vi "Main VI.vi"(8 "error in":errorcluster) -> (0 "error out":errorcluster)   [LabVIEW 2023, in "Decoder.lvlib"]
uses:
  Decoder.lvlib
  <vilib>/xnet/xnet.llb/XNET Frame CAN.ctl
  <vilib>/xnet/xnet.llb/XNET Frame Type CAN.ctl
  <vilib>/xnet/xnet.llb/XNET Create Session (Frame Input Single-point).vi
  <vilib>/xnet/xnet.llb/XNET Read (Frame CAN).vi
  Internal Communication/Internal Communication.lvlib
  FPGA/FPGA.lvlib
panel:
  in  "x":bool
  out "Boolean":bool
  out "x != y?":bool
  out "element":T1 {"payload" format="%x"; "timestamp" format="%<%.7X\n%x>T"; "type" items=["CAN Data"=0, "CAN Remote"=1, "CAN Bus Error"=2, "CAN 2.0 Data"=8, "CAN FD Data"=16, "CAN FD+BRS Data"=24, "J1939 Data"=192, "Delay"=224, "Log Trigger"=225, "Start Trigger"=226]; "identifier" format="%x"}
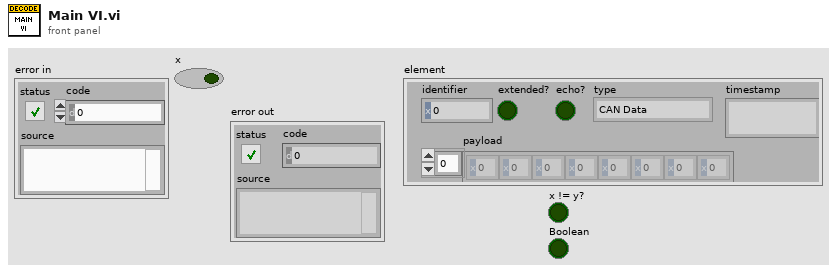
[diagram p1: front panel]
types:
  T1 = typedef "XNET Frame CAN.ctl" = cluster{"timestamp":timestamp, "payload":u8[], "identifier":u32, "type":T2, "extended?":bool, "echo?":bool}
  T2 = typedef "XNET Frame Type CAN.ctl" = u8
  T3 = typedef "Queue.ctl" = refnum<queue>
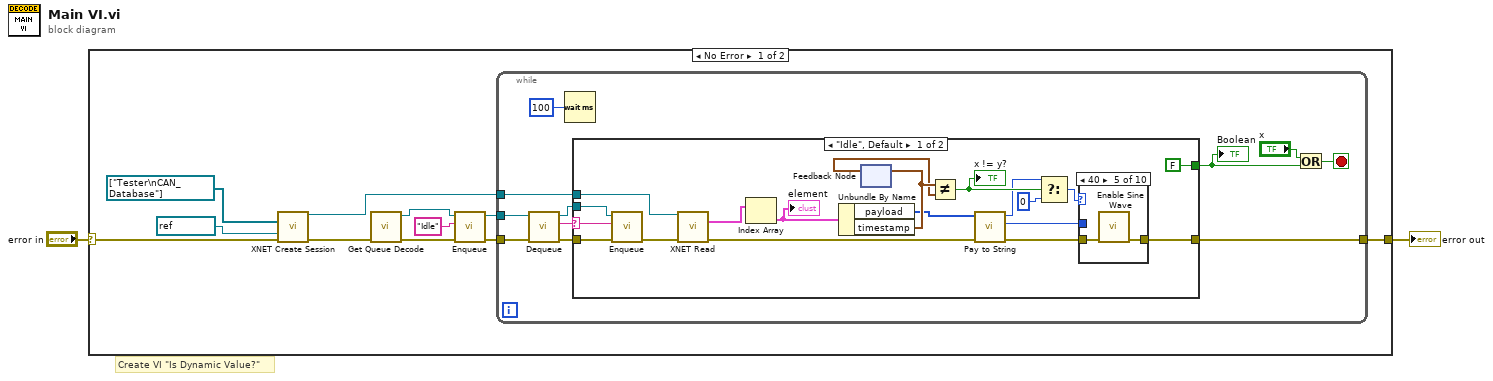
[diagram p0: block diagram]
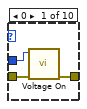
[diagram p2: hidden frame]
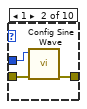
[diagram p3: hidden frame]
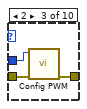
[diagram p4: hidden frame]
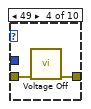
[diagram p5: hidden frame]
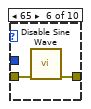
[diagram p6: hidden frame]
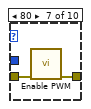
[diagram p7: hidden frame]
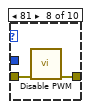
[diagram p8: hidden frame]
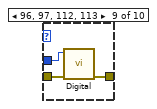
[diagram p9: hidden frame]
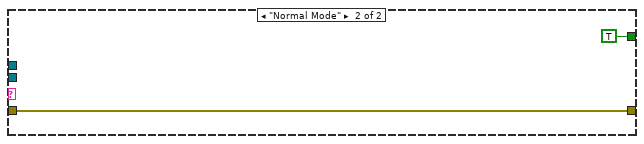
[diagram p11: hidden frame]
diagram:
  # "Create VI \"Is Dynamic Value?\""
  n1 = case shown="No Error" "error in" {
    selector: "error in" -> [w3 w69]
    tunnel: [w13 w69] -> w2
    frame No Error {
      n2 = call-poly <vilib>:"XNET Create Session.vi"("frame list"=refnum<k21>[] ["Tester\nCAN_Database"], "interface"=refnum<k21> "CAN2", "error in (no error)"=w3) -> ("session out"=w10:refnum<k21>, "error out"=w6:errorcluster)  [unwired: 11 in]
      n3 = call "Get Queue Decode.vi"("error in (no error)"=w6) -> ("error out"=w8:errorcluster, "Decoder Queue"=w9:refnum<queue>)  [unwired: 9 in]
      n4 = call "Enqueue.vi"("error in (no error)"=w8, "Command"="Idle", "Queue In"=w9) -> ("error out"=w5:errorcluster, "Queue Out"=w4:T3)  [unwired: 7 in]
      n5 = while {
        tunnel: w10 -> [w24]
        tunnel: w5 -> [w21]
        tunnel: [w23] -> w13
        tunnel: w4 -> [w19]
        stop <- w17 stop-if-true
        n6 = call "Dequeue.vi"("error in (no error)"=w21, "Queue In"=w19) -> ("error out"=w20:errorcluster, "String"=w18:string, "Queue Out"=w14:T3)  [unwired: 6 in, 1 out]
        n7 = Wait (ms)(milliseconds to wait=u32 100) -> ()  [unwired: 1 out]
        n8 = case shown="\"Idle\", Default" w18 {
          selector: w18 -> [w35 _]
          tunnel: [FALSE ("Boolean") TRUE ("Boolean 2")] -> w16
          tunnel: w24 -> [w43 _]
          tunnel: [w26 w67] -> w23
          tunnel: w20 -> [w37 w67]
          tunnel: w14 -> [w36 _]
          frame "Idle", Default {
            n9 = call "Enqueue.vi"("error in (no error)"=w37, "Command"=w35, "Queue In"=w36) -> ("error out"=w34:errorcluster)  [unwired: 7 in, 1 out]
            n10 = call-poly <vilib>:"XNET Read.vi"("session in"=w43, "error in (no error)"=w34) -> ("data"=w42:T1[], "error out"=w30:errorcluster)  [unwired: 12 out]
            n11 = Index Array(array=w42) -> (element=w39:T1)  [unwired: 1 in]
            "element" <- w39
            n12 = Unbundle By Name(w39) -> ("payload"=w32:u8[], "timestamp"=w41:timestamp)
            n13 = feedback #1() -> (w40:timestamp)  [unwired: 1 in]
            n14 = feedback-in #1(w41) -> ()
            n15 = Not Equal?(x=w41, y=w40) -> (x != y?=w33:bool)
            "x != y?" <- w33
            n16 = call "Pay to String.vi"("error in"=w30, "payload"=w32) -> ("error out"=w27:errorcluster, "Extra Value"=w25:u8, "State"=w31:u8)  [unwired: 7 in]
            n17 = Select(t=w31, s=w33, f=u8 0) -> (s? t:f=w29:u8)
            n18 = case shown="40" w29 {
              tunnel: w27 -> [w46 w49 w51 w54 w56 w58 w60 w62 w65 w66]
              tunnel: [w45 w48 w52 w53 w55 w57 w59 w61 w64 w66] -> w26
              tunnel: w25 -> [w44 w47 w50 _ _ _ _ _ w63 _]
              frame 0 {
                n19 = call "Voltage On.vi"("error in (no error)"=w46, "Data"=w44) -> ("error out"=w45:errorcluster)  [unwired: 8 in, 1 out]
              }
              frame 1 {
                n20 = call "Config Sine Wave.vi"("error in (no error)"=w49, "Data"=w47) -> ("error out"=w48:errorcluster)  [unwired: 9 in]
              }
              frame 2 {
                n21 = call "Config PWM.vi"("error in (no error)"=w51, "Data"=w50) -> ("error out"=w52:errorcluster)  [unwired: 9 in]
              }
              frame 49 {
                n22 = call "Voltage Off.vi"("error in (no error)"=w54) -> ("error out"=w53:errorcluster)  [unwired: 9 in, 1 out]
              }
              frame 64 {
                n23 = call "Enable Sine Wave.vi"("error in (no error)"=w56) -> ("error out"=w55:errorcluster)  [unwired: 10 in]
              }
              frame 65 {
                n24 = call "Disable Sine Wave.vi"("error in (no error)"=w58) -> ("error out"=w57:errorcluster)  [unwired: 10 in]
              }
              frame 80 {
                n25 = call "Enable PWM.vi"("error in (no error)"=w60) -> ("error out"=w59:errorcluster)  [unwired: 10 in]
              }
              frame 81 {
                n26 = call "Disable PWM.vi"("error in (no error)"=w62) -> ("error out"=w61:errorcluster)  [unwired: 10 in]
              }
              frame 96, 97, 112, 113 {
                n27 = call "Digital.vi"("error in (no error)"=w65, "Data"=w63) -> ("error out"=w64:errorcluster)  [unwired: 9 in]
              }
              frame 105, Default {
              }
            }
          }
          frame "Normal Mode" {
          }
        }
        "Boolean" <- w16
        n28 = Or(x="x", y=w16) -> (x .or. y?=w17:bool)
      }
    }
    frame Error {
    }
  }
  "error out" <- w2
